vi "UpdateFFTwindow.vi"(9 "subwindow IN":T2={"2^n : x"=10, "2^n : y"=10, "lower left box Position"={"X"=1752.0, "Y"=1167.0}, "Height"=0, "Width"=0} {"Width" min=32 max=4704; "Height" min=2 max=3424; "2^n : y" min=1 max=13; "2^n : x" min=1 max=13}, 11 "Intensity Graph":refnum<vi>) -> (2 "output cluster":T1)   [LabVIEW 2018]
uses:
  <vilib>/Utility/miscctls.llb/LVPointDoubleTypeDef.ctl
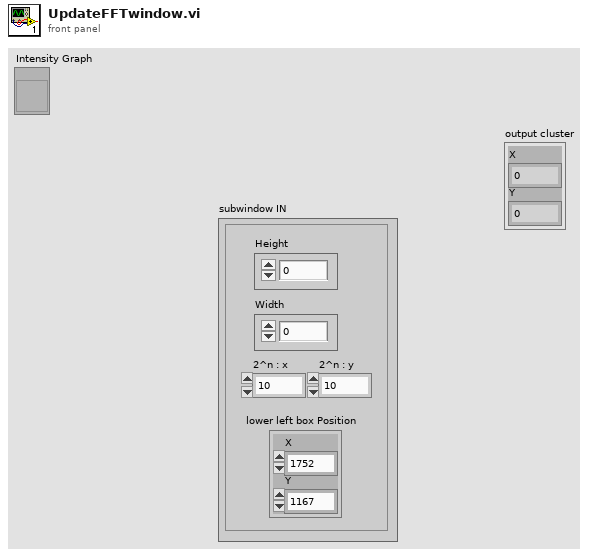
[diagram p1: front panel]
types:
  T1 = typedef "LVPointDoubleTypeDef.ctl" = cluster{"X":dbl, "Y":dbl}
  T2 = cluster{"2^n : x":i8, "2^n : y":i8, "lower left box Position":T1, "Height":i32, "Width":i32}
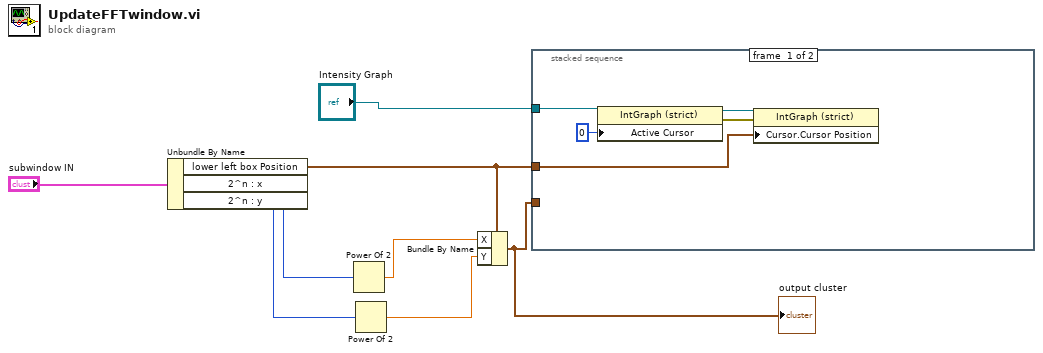
[diagram p0: block diagram]
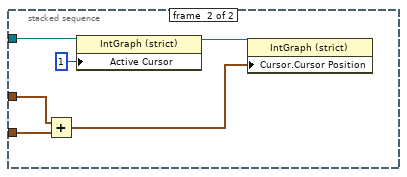
[diagram p2: hidden frame]
diagram:
  n1 = Unbundle By Name("subwindow IN") -> ("lower left box Position"=w6:T1, "2^n : x"=w8:i8, "2^n : y"=w7:i8)
  n2 = Power Of 2(x=w8) -> (2^x=w5:dbl)
  n3 = Power Of 2(x=w7) -> (2^x=w4:dbl)
  n4 = Bundle By Name(cluster=w6, "X"=w5, "Y"=w4) -> (w3:T1)
  "output cluster" <- w3
  n5 = stacked-sequence {
    tunnel: "Intensity Graph" -> [w13 w19]
    tunnel: w6 -> [w10 w15]
    tunnel: w3 -> [_ w16]
    frame #0 {
      n6 = property class="IntGraph (strict)"(reference=w13, "Active Cursor"=u32 0) -> (reference out=w11:refnum<vi>, error out=w9:errorcluster)  [unwired: 1 in]
      n7 = property class="IntGraph (strict)"(reference=w11, error in=w9, "Cursor.Cursor Position"=w10) -> ()  [unwired: 2 out]
    }
    frame #1 {
      n8 = Add(x=w15, y=w16) -> (x+y=w14:T1)
      n9 = property class="IntGraph (strict)"(reference=w19, "Active Cursor"=u32 1) -> (reference out=w17:refnum<vi>)  [unwired: 1 in, 1 out]
      n10 = property class="IntGraph (strict)"(reference=w17, "Cursor.Cursor Position"=w14) -> ()  [unwired: 1 in, 2 out]
    }
  }
